vi "GetCameraByName.vi"(10 "name":string, 11 "cameras in":T1[](array[typedef])) -> (1 "found":bool, 2 "camera":T1, 3 "cameras out":T1[](array[typedef]))   [LabVIEW 2017, in "DeviceModelHelpers.lvlib"]
uses:
  <vilib>/addons/InsightCM/Utilities/DeviceModelHelpers/DeviceModelHelpers.lvlib
  <vilib>/addons/InsightCM/MessageBus/Base/controls/Camera.ctl
  <vilib>/addons/InsightCM/MessageBus/Base/controls/KeyValuePair.ctl
  <vilib>/addons/InsightCM/MessageBus/Base/controls/Trigger.ctl
  <vilib>/addons/InsightCM/MessageBus/Base/controls/Condition.ctl
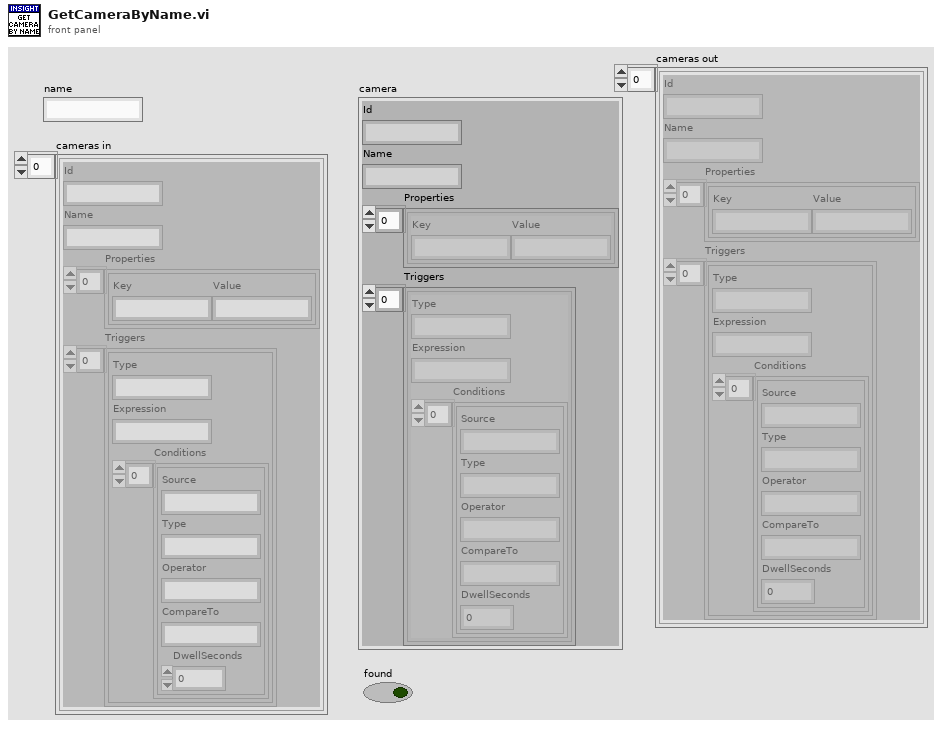
[diagram p1: front panel]
types:
  T1 = typedef "Camera.ctl" = cluster{"Id":string, "Name":string, "Properties":T2[], "Triggers":T3[]}
  T2 = typedef "KeyValuePair.ctl" = cluster{"Key":string, "Value":string}
  T3 = typedef "Trigger.ctl" = cluster{"Type":string, "Expression":string, "Conditions":T4[]}
  T4 = typedef "Condition.ctl" = cluster{"Source":string, "Type":string, "Operator":string, "CompareTo":string, "DwellSeconds":dbl}
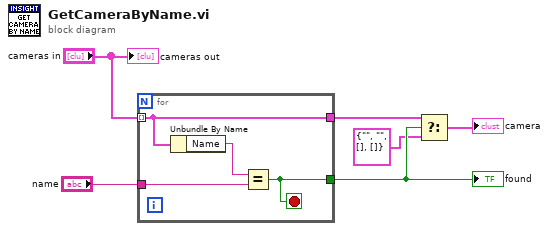
[diagram p0: block diagram]
diagram:
  n1 = for {
    tunnel: "cameras in" -> [w8] mode=indexing
    tunnel: "name" -> [w9]
    tunnel: [w8] -> w4
    tunnel: [w7] -> w2
    stop <- w7 stop-if-true
    n2 = Unbundle By Name(w8) -> ("Name"=w10:string)
    n3 = Equal?(x=w10, y=w9) -> (x = y?=w7:bool)
  }
  "found" <- w2
  n4 = Select(t=w4, s=w2, f=T1 {"Id"="", "Name"="", "Properties"=[], "Triggers"=[]} ("camera")) -> (s? t:f=→"camera":T1)
  "cameras out" <- "cameras in"
